vi "Read state.vi"(8 "error in (no error)":errorcluster, 11 "Change Speaker State CMD in":refnum<class "Change Filter State CMD.lvclass">) -> (0 "error out":errorcluster, 2 "state":bool, 3 "Change Speaker State CMD out":refnum<class "Change Filter State CMD.lvclass">)   [LabVIEW 2017, in "PAS Library.lvlib" / "Change Filter State CMD.lvclass"]
uses:
  Change Filter State CMD.lvclass
  Change Filter State CMD.lvclass/Change Filter State CMD.ctl
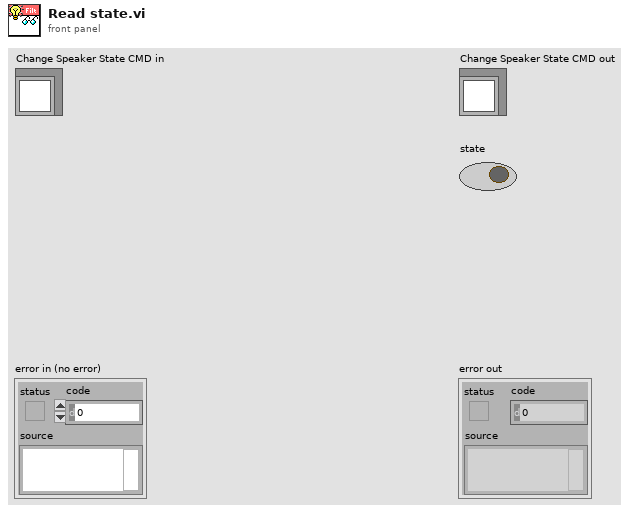
[diagram p1: front panel]
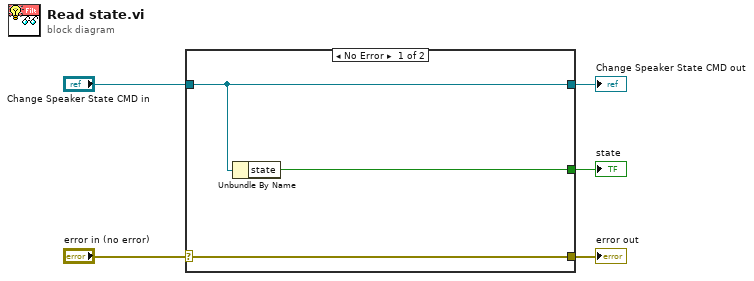
[diagram p0: block diagram]
diagram:
  n1 = case shown="No Error" "error in (no error)" {
    selector: "error in (no error)" -> [w8 w9]
    tunnel: [w8 w9] -> w4
    tunnel: [w7 w10] -> w2
    tunnel: "Change Speaker State CMD in" -> [w7 w10]
    tunnel: [w6 _] -> w1
    frame No Error {
      n2 = Unbundle By Name(w7) -> ("state"=w6:bool)
    }
    frame Error {
    }
  }
  "error out" <- w4
  "Change Speaker State CMD out" <- w2
  "state" <- w1
